vi "Read DVR_voltage.vi"(8 "error in (no error)":errorcluster, 11 "command_parser in":refnum<class "command_parser.lvclass">) -> (0 "error out":errorcluster, 2 "DVR_voltage":refnum<data-value>, 3 "command_parser out":refnum<class "command_parser.lvclass">)   [LabVIEW 2025, in "command_parser.lvlib" / "command_parser.lvclass"]
uses:
  command_parser.lvclass
  command_parser.lvclass/command_parser.ctl
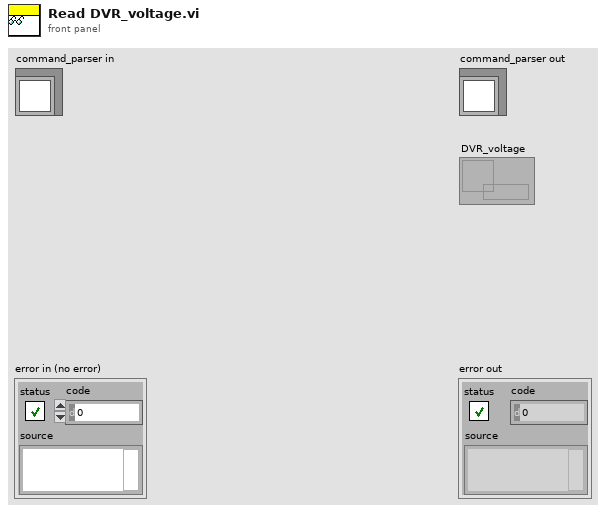
[diagram p1: front panel]
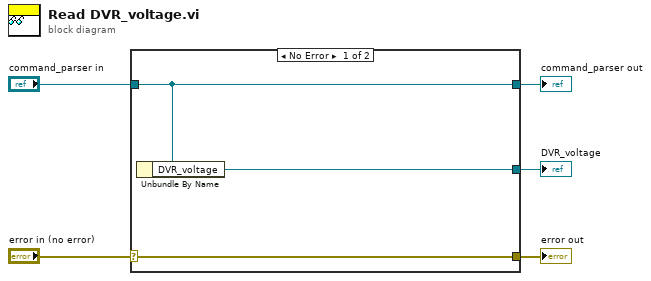
[diagram p0: block diagram]
diagram:
  n1 = case shown="No Error" "error in (no error)" {
    selector: "error in (no error)" -> [w8 w9]
    tunnel: [w8 w9] -> w4
    tunnel: [w7 w10] -> w2
    tunnel: "command_parser in" -> [w7 w10]
    tunnel: [w6 _] -> w1
    frame No Error {
      n2 = Unbundle By Name(w7) -> ("DVR_voltage"=w6:refnum<data-value>)
    }
    frame Error {
    }
  }
  "error out" <- w4
  "command_parser out" <- w2
  "DVR_voltage" <- w1
